vi "LEDSineGenerator.vi"(9 "Amplitude":dbl, 10 "Speed":dbl, 11 "Delay":dbl) -> (2 "Output":dbl)   [LabVIEW 2023]
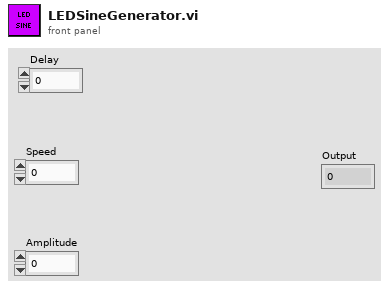
[diagram p1: front panel]
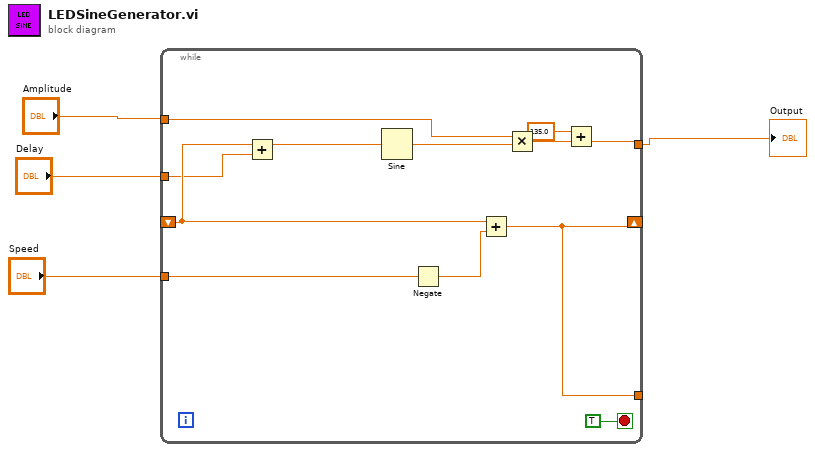
[diagram p0: block diagram]
diagram:
  n1 = while {
    shift-right: [w14] -> _
    shift-left: _ -> [w15]
    tunnel: [w6] -> w1
    tunnel: [w14] -> _
    tunnel: "Delay" -> [w10]
    tunnel: "Speed" -> [w9]
    tunnel: "Amplitude" -> [w8]
    stop <- TRUE stop-if-true
    n2 = Add(x=w15, y=w10) -> (x+y=w11:dbl)
    n3 = Sine(x=w11) -> (sin(x)=w13:dbl)
    n4 = Negate(x=w9) -> (-x=w7:dbl)
    n5 = Add(x=w15, y=w7) -> (x+y=w14:dbl)
    n6 = Multiply(x=w8, y=w13) -> (x*y=w12:dbl)
    n7 = Add(x=135.0, y=w12) -> (x+y=w6:dbl)
  }
  "Output" <- w1
